vi "Add Status Sections.vi"(8 "error in (no error)":errorcluster, 11 "Item Ref in":T1 format="%.0x") -> (0 "error out":errorcluster, 3 "Item Ref out":T1 format="%.0x")   [LabVIEW 2019]
uses:
  DSF System Explorer.lvlib
  Shared/DSF Shared.lvlib
  Shared/Plugin Page GUID.vi
  Shared/Transfer Page GUID.vi
  <vilib>/NI VeriStand/Custom Device API/Custom Device Item Ref.ctl
  <vilib>/NI VeriStand/Custom Device API/Custom Device API.lvlib
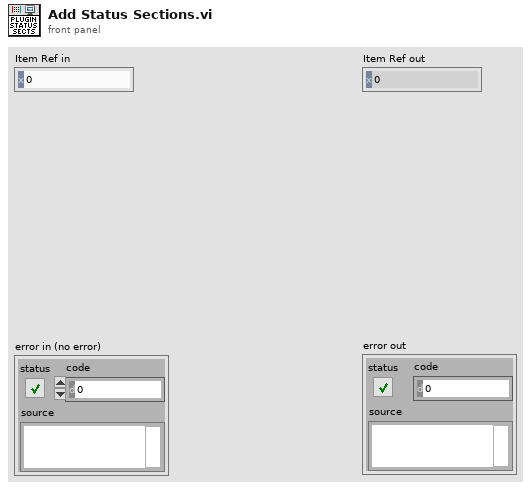
[diagram p1: front panel]
types:
  T1 = typedef "Custom Device API.lvlib/Custom Device Item Ref.ctl" = u64
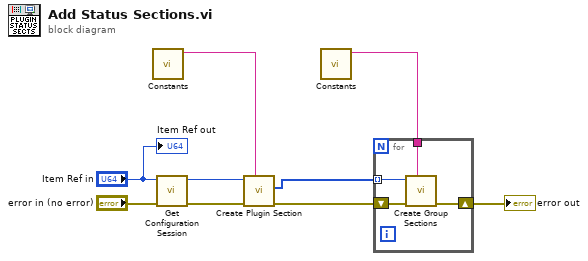
[diagram p0: block diagram]
diagram:
  n1 = call-poly "Constants.vi"() -> ("Plugin GUID"=w2:string)  [unwired: 11 in]
  n2 = call "Get Configuration Session.vi"("error in (no error)"="error in (no error)", "Item Ref in"="Item Ref in") -> ("error out"=w8:errorcluster, "Item Ref out"=w7:T1)  [unwired: 7 in, 1 out]
  n3 = call "Create Plugin Section.vi"("GUID (Default Section)"=w2, "error in (no error)"=w8, "Item Ref in"=w7) -> ("error out"=w6:errorcluster, "Plugin Section refs"=w5:T1[])  [unwired: 6 in, 1 out]
  n4 = call-poly "Constants.vi"() -> ("Transfer GUID"=w1:string)  [unwired: 11 in]
  n5 = for {
    shift-right: [w11] -> w3
    shift-left: w6 -> [w13]
    tunnel: w5 -> [w12] mode=indexing
    tunnel: w1 -> [w10]
    n6 = call "Create Group Sections.vi"("GUID (Default Section)"=w10, "error in (no error)"=w13, "Item Ref in"=w12) -> ("error out"=w11:errorcluster)  [unwired: 6 in, 2 out]
  }
  "error out" <- w3
  "Item Ref out" <- "Item Ref in"
